vi "Get md5 with MAC.vi"(8 "error in (no error)":errorcluster, 11 "prefix text":string="tctechinc") -> (0 "error out":errorcluster, 3 "MD5 Message Digest":string)   [LabVIEW 2016]
panel:
  out "MAC address":string
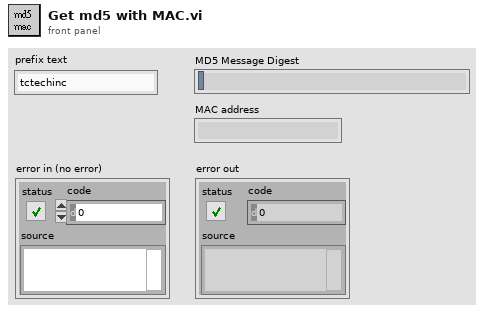
[diagram p1: front panel]
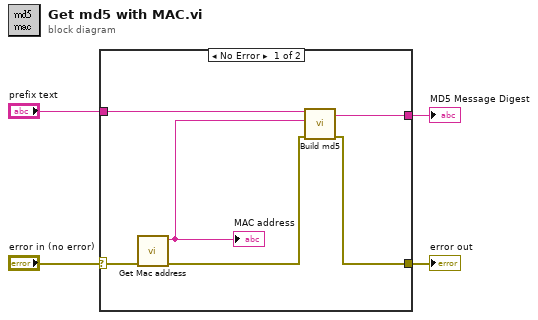
[diagram p0: block diagram]
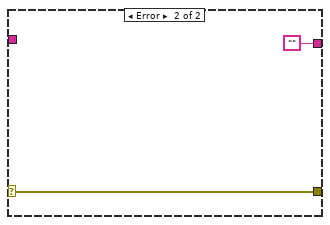
[diagram p2: hidden frame]
diagram:
  n1 = case shown="No Error" "error in (no error)" {
    selector: "error in (no error)" -> [w7 w12]
    tunnel: [w10 ""] -> w4
    tunnel: "prefix text" -> [w9 _]
    tunnel: [w5 w12] -> w1
    frame No Error {
      n2 = call "Get Mac address.vi"("error in (no error)"=w7) -> ("error out"=w6:errorcluster, "MAC address"=w8:string)  [unwired: 9 in]
      "MAC address" <- w8
      n3 = call "Build md5.vi"("error in (no error)"=w6, "words"=w8, "prefix"=w9) -> ("error out"=w5:errorcluster, "MD5 Message Digest"=w10:string)  [unwired: 7 in]
    }
    frame Error {
    }
  }
  "MD5 Message Digest" <- w4
  "error out" <- w1
